vi "canDataSort.vi"() -> ()   [LabVIEW 2023] (continued)
database", "NameShort"="BMS06BattMinTempPoint2", "StartBit"=16, "NumBits"=8, "Min"=-40.0, "Max"=210.0, "ScaleFac"=1.0, "ScaleOff"=-40.0}, {"18F142F3", "Frame"="BMS06\ndatabase", "NameShort"="BMS06BattMinTempPoint2BoxNum", "StartBit"=24, "NumBits"=8, "Min"=0.0, "Max"=100.0, "ScaleFac"=1.0, "ScaleOff"=0.0}, {"18F142F3", "Frame"="BMS06\ndatabase", "NameShort"="BMS06BattMinTempPoint3", "StartBit"=32, "NumBits"=8, "Min"=-40.0, "Max"=210.0, "ScaleFac"=1.0, "ScaleOff"=-40.0}, {"18F142F3", "Frame"="BMS06\ndatabase", "NameShort"="BMS06BattMinTempPoint3BoxNum", "StartBit"=40, "NumBits"=8, "Min"=0.0, "Max"=100.0, "ScaleFac"=1.0, "ScaleOff"=0.0}, {"18F142F3", "Frame"="BMS06\ndatabase", "NameShort"="BMS06BattMinTempPoint4", "StartBit"=48, "NumBits"=8, "Min"=-40.0, "Max"=210.0, "ScaleFac"=1.0, "ScaleOff"=-40.0}, {"18F142F3", "Frame"="BMS06\ndatabase", "NameShort"="BMS06BattMinTempPoint4BoxNum", "StartBit"=56, "NumBits"=8, "Min"=0.0, "Max"=100.0, "ScaleFac"=1.0, "ScaleOff"=0.0}, {"18F143F3", "Frame"="BMS07\ndatabase", "NameShort"="BMS06BattMaxTempPoint1", "StartBit"=0, "NumBits"=8, "Min"=-40.0, "Max"=210.0, "ScaleFac"=1.0, "ScaleOff"=-40.0}, {"18F143F3", "Frame"="BMS07\ndatabase", "NameShort"="BMS06BattMaxTempPoint1BoxNum", "StartBit"=8, "NumBits"=8, "Min"=0.0, "Max"=100.0, "ScaleFac"=1.0, "ScaleOff"=0.0}, {"18F143F3", "Frame"="BMS07\ndatabase", "NameShort"="BMS06BattMaxTempPoint2", "StartBit"=16, "NumBits"=8, "Min"=-40.0, "Max"=210.0, "ScaleFac"=1.0, "ScaleOff"=-40.0}, {"18F143F3", "Frame"="BMS07\ndatabase", "NameShort"="BMS06BattMaxTempPoint2BoxNum", "StartBit"=24, "NumBits"=8, "Min"=0.0, "Max"=100.0, "ScaleFac"=1.0, "ScaleOff"=0.0}, {"18F143F3", "Frame"="BMS07\ndatabase", "NameShort"="BMS06BattMaxTempPoint3", "StartBit"=32, "NumBits"=8, "Min"=-40.0, "Max"=210.0, "ScaleFac"=1.0, "ScaleOff"=-40.0}, {"18F143F3", "Frame"="BMS07\ndatabase", "NameShort"="BMS06BattMaxTempPoint3BoxNum", "StartBit"=40, "NumBits"=8, "Min"=0.0, "Max"=100.0, "ScaleFac"=1.0, "ScaleOff"=0.0}, {"18F143F3", "Frame"="BMS07\ndatabase", "NameShort"="BMS06BattMaxTempPoint4", "StartBit"=48, "NumBits"=8, "Min"=-40.0, "Max"=210.0, "ScaleFac"=1.0, "ScaleOff"=-40.0}, {"18F143F3", "Frame"="BMS07\ndatabase", "NameShort"="BMS06BattMaxTempPoint4BoxNum", "StartBit"=56, "NumBits"=8, "Min"=0.0, "Max"=100.0, "ScaleFac"=1.0, "ScaleOff"=0.0}, {"18F144F3", "Frame"="BMS08\ndatabase", "NameShort"="BMS08BattCellMinVolt1", "StartBit"=0, "NumBits"=16, "Min"=0.0, "Max"=655.35, "ScaleFac"=0.01, "ScaleOff"=0.0}, {"18F144F3", "Frame"="BMS08\ndatabase", "NameShort"="BMS08BattCellMinVolt1Box", "StartBit"=24, "NumBits"=8, "Min"=0.0, "Max"=255.0, "ScaleFac"=1.0, "ScaleOff"=0.0}, {"18F144F3", "Frame"="BMS08\ndatabase", "NameShort"="BMS08BattCellMinVolt1Num", "StartBit"=16, "NumBits"=8, "Min"=0.0, "Max"=100.0, "ScaleFac"=1.0, "ScaleOff"=0.0}, {"18F144F3", "Frame"="BMS08\ndatabase", "NameShort"="BMS08BattCellMinVolt2", "StartBit"=32, "NumBits"=16, "Min"=0.0, "Max"=655.35, "ScaleFac"=0.01, "ScaleOff"=0.0}, {"18F144F3", "Frame"="BMS08\ndatabase", "NameShort"="BMS08BattCellMinVolt2Box", "StartBit"=56, "NumBits"=8, "Min"=0.0, "Max"=255.0, "ScaleFac"=1.0, "ScaleOff"=0.0}, {"18F144F3", "Frame"="BMS08\ndatabase", "NameShort"="BMS08BattCellMinVolt2Num", "StartBit"=48, "NumBits"=8, "Min"=0.0, "Max"=100.0, "ScaleFac"=1.0, "ScaleOff"=0.0}, {"18F145F3", "Frame"="BMS09\ndatabase", "NameShort"="BMS09BattCellMinVolt3", "StartBit"=0, "NumBits"=16, "Min"=0.0, "Max"=655.35, "ScaleFac"=0.01, "ScaleOff"=0.0}, {"18F145F3", "Frame"="BMS09\ndatabase", "NameShort"="BMS09BattCellMinVolt3Box", "StartBit"=24, "NumBits"=8, "Min"=0.0, "Max"=255.0, "ScaleFac"=1.0, "ScaleOff"=0.0}, {"18F145F3", "Frame"="BMS09\ndatabase", "NameShort"="BMS09BattCellMinVolt3Num", "StartBit"=16, "NumBits"=8, "Min"=0.0, "Max"=100.0, "ScaleFac"=1.0, "ScaleOff"=0.0}, {"18F145F3", "Frame"="BMS09\ndatabase", "NameShort"="BMS09BattCellMinVolt4", "StartBit"=32, "NumBits"=16, "Min"=0.0, "Max"=655.35, "ScaleFac"=0.01, "ScaleOff"=0.0}, {"18F145F3", "Frame"="BMS09\ndatabase", "NameShort"="BMS09BattCellMinVolt4Box", "StartBit"=56, "NumBits"=8, "Min"=0.0, "Max"=255.0, "ScaleFac"=1.0, "ScaleOff"=0.0}, {"18F145F3", "Frame"="BMS09\ndatabase", "NameShort"="BMS09BattCellMinVolt4Num", "StartBit"=48, "NumBits"=8, "Min"=0.0, "Max"=100.0, "ScaleFac"=1.0, "ScaleOff"=0.0}, {"18F146F3", "Frame"="BMS10\ndatabase", "NameShort"="BMS10BattCellMinVolt1", "StartBit"=0, "NumBits"=16, "Min"=0.0, "Max"=655.35, "ScaleFac"=0.01, "ScaleOff"=0.0}, {"18F146F3", "Frame"="BMS10\ndatabase", "NameShort"="BMS10BattCellMinVolt1Box", "StartBit"=24, "NumBits"=8, "Min"=0.0, "Max"=255.0, "ScaleFac"=1.0, "ScaleOff"=0.0}, {"18F146F3", "Frame"="BMS10\ndatabase", "NameShort"="BMS10BattCellMinVolt1Num", "StartBit"=16, "NumBits"=8, "Min"=0.0, "Max"=100.0, "ScaleFac"=1.0, "ScaleOff"=0.0}, {"18F146F3", "Frame"="BMS10\ndatabase", "NameShort"="BMS10BattCellMinVolt2", "StartBit"=32, "NumBits"=16, "Min"=0.0, "Max"=655.35, "ScaleFac"=0.01, "ScaleOff"=0.0}, {"18F146F3", "Frame"="BMS10\ndatabase", "NameShort"="BMS10BattCellMinVolt2Box", "StartBit"=56, "NumBits"=8, "Min"=0.0, "Max"=255.0, "ScaleFac"=1.0, "ScaleOff"=0.0}, {"18F146F3", "Frame"="BMS10\ndatabase", "NameShort"="BMS10BattCellMinVolt2Num", "StartBit"=48, "NumBits"=8, "Min"=0.0, "Max"=100.0, "ScaleFac"=1.0, "ScaleOff"=0.0}, {"18F147F3", "Frame"="BMS11\ndatabase", "NameShort"="BMS11BattCellMinVolt3", "StartBit"=0, "NumBits"=16, "Min"=0.0, "Max"=655.35, "ScaleFac"=0.01, "ScaleOff"=0.0}, {"18F147F3", "Frame"="BMS11\ndatabase", "NameShort"="BMS11BattCellMinVolt3Box", "StartBit"=24, "NumBits"=8, "Min"=0.0, "Max"=255.0, "ScaleFac"=1.0, "ScaleOff"=0.0}, {"18F147F3", "Frame"="BMS11\ndatabase", "NameShort"="BMS11BattCellMinVolt3Num", "StartBit"=16, "NumBits"=8, "Min"=0.0, "Max"=100.0, "ScaleFac"=1.0, "ScaleOff"=0.0}, {"18F147F3", "Frame"="BMS11\ndatabase", "NameShort"="BMS11BattCellMinVolt4", "StartBit"=32, "NumBits"=16, "Min"=0.0, "Max"=655.35, "ScaleFac"=0.01, "ScaleOff"=0.0}, {"18F147F3", "Frame"="BMS11\ndatabase", "NameShort"="BMS11BattCellMinVolt4Box", "StartBit"=56, "NumBits"=8, "Min"=0.0, "Max"=255.0, "ScaleFac"=1.0, "ScaleOff"=0.0}, {"18F147F3", "Frame"="BMS11\ndatabase", "NameShort"="BMS11BattCellMinVolt4Num", "StartBit"=48, "NumBits"=8, "Min"=0.0, "Max"=100.0, "ScaleFac"=1.0, "ScaleOff"=0.0}, {"18F148F3", "Frame"="BMS12\ndatabase", "NameShort"="BMS12BattPackProdMonth", "StartBit"=40, "NumBits"=8, "Min"=0.0, "Max"=12.0, "ScaleFac"=1.0, "ScaleOff"=0.0}, {"18F148F3", "Frame"="BMS12\ndatabase", "NameShort"="BMS12BattPackProdYear", "StartBit"=32, "NumBits"=8, "Min"=1985.0, "Max"=2235.0, "ScaleFac"=1.0, "ScaleOff"=1985.0}, {"18F148F3", "Frame"="BMS12\ndatabase", "NameShort"="BMS12BattProdDay", "StartBit"=48, "NumBits"=8, "Min"=0.0, "Max"=31.0, "ScaleFac"=1.0, "ScaleOff"=0.0}, {"18F148F3", "Frame"="BMS12\ndatabase", "NameShort"="BMS12BattRatedCapacity", "StartBit"=0, "NumBits"=16, "Min"=0.0, "Max"=1000.0, "ScaleFac"=1.0, "ScaleOff"=0.0}, {"18F148F3", "Frame"="BMS12\ndatabase", "NameShort"="BMS12BattRatedVolt", "StartBit"=16, "NumBits"=16, "Min"=0.0, "Max"=1000.0, "ScaleFac"=1.0, "ScaleOff"=0.0}, {"18FFC3A9", "Frame"="BluestarAirConErrorNBoot\ndatabase", "NameShort"="BluestarAirConElectricBoxPow", "StartBit"=40, "NumBits"=2, "Min"=0.0, "Max"=2.0, "ScaleFac"=1.0, "ScaleOff"=0.0}, {"18FFC3A9", "Frame"="BluestarAirConErrorNBoot\ndatabase", "NameShort"="BluestarAirConErr01Overvoltage", "StartBit"=4, "NumBits"=2, "Min"=0.0, "Max"=1.0, "ScaleFac"=1.0, "ScaleOff"=0.0}, {"18FFC3A9", "Frame"="BluestarAirConErrorNBoot\ndatabase", "NameShort"="BluestarAirConErr02Undervoltage", "StartBit"=6, "NumBits"=2, "Min"=0.0, "Max"=1.0, "ScaleFac"=1.0, "ScaleOff"=0.0}, {"18FFC3A9", "Frame"="BluestarAirConErrorNBoot\ndatabase", "NameShort"="BluestarAirConErr03UnderPressure", "StartBit"=0, "NumBits"=2, "Min"=0.0, "Max"=2.0, "ScaleFac"=1.0, "ScaleOff"=0.0}, {"18FFC3A9", "Frame"="BluestarAirConErrorNBoot\ndatabase", "NameShort"="BluestarAirConErr04EDefroster", "StartBit"=14, "NumBits"=2, "Min"=0.0, "Max"=2.0, "ScaleFac"=1.0, "ScaleOff"=0.0}, {"18FFC3A9", "Frame"="BluestarAirConErrorNBoot\ndatabase", "NameShort"="BluestarAirConErr05IndoorSensor", "StartBit"=8, "NumBits"=2, "Min"=0.0, "Max"=2.0, "ScaleFac"=1.0, "ScaleOff"=0.0}, {"18FFC3A9", "Frame"="BluestarAirConErrorNBoot\ndatabase", "NameShort"="BluestarAirConErr07OverPressure", "StartBit"=2, "NumBits"=2, "Min"=0.0, "Max"=2.0, "ScaleFac"=1.0, "ScaleOff"=0.0}, {"18FFC3A9", "Frame"="BluestarAirConErrorNBoot\ndatabase", "NameShort"="BluestarAirConErr08OutdoorSensor", "StartBit"=10, "NumBits"=2, "Min"=0.0, "Max"=2.0, "ScaleFac"=1.0, "ScaleOff"=0.0}, {"18FFC3A9", "Frame"="BluestarAirConErrorNBoot\ndatabase", "NameShort"="BluestarAirConErr09Compressor", "StartBit"=32, "NumBits"=2, "Min"=0.0, "Max"=2.0, "ScaleFac"=1.0, "ScaleOff"=0.0}, {"18FFC3A9", "Frame"="BluestarAirConErrorNBoot\ndatabase", "NameShort"="BluestarAirConErr10Inverter", "StartBit"=28, "NumBits"=2, "Min"=0.0, "Max"=2.0, "ScaleFac"=1.0, "ScaleOff"=0.0}, {"18FFC2A9", "Frame"="BluestarAirConRemotePowerContro2\ndatabase", "NameShort"="BluestarAirConIndoorTemp", "StartBit"=0, "NumBits"=8, "Min"=-40.0, "Max"=210.0, "ScaleFac"=1.0, "ScaleOff"=-40.0}, {"18FFC2A9", "Frame"="BluestarAirConRemotePowerContro2\ndatabase", "NameShort"="BluestarAirConOutdoorTemp", "StartBit"=8, "NumBits"=8, "Min"=-40.0, "Max"=210.0, "ScaleFac"=1.0, "ScaleOff"=-40.0}, {"18FFC1A8", "Frame"="BluestarAirConRemotePowerControl\ndatabase", "NameShort"="BluestarAirConAutoMode", "StartBit"=44, "NumBits"=2, "Min"=0.0, "Max"=1.0, "ScaleFac"=1.0, "ScaleOff"=0.0}, {"18FFC1A8", "Frame"="BluestarAirConRemotePowerControl\ndatabase", "NameShort"="BluestarAirConFanSpeed", "StartBit"=4, "NumBits"=4, "Min"=0.0, "Max"=1.0, "ScaleFac"=1.0, "ScaleOff"=0.0}, {"18FFC1A8", "Frame"="BluestarAirConRemotePowerControl\ndatabase", "NameShort"="BluestarAirConMode", "StartBit"=8, "NumBits"=8, "Min"=0.0, "Max"=1.0, "ScaleFac"=1.0, "ScaleOff"=0.0}, {"18FFC1A8", "Frame"="BluestarAirConRemotePowerControl\ndatabase", "NameShort"="BluestarAirConPowerOnOff", "StartBit"=0, "NumBits"=2, "Min"=0.0, "Max"=1.0, "ScaleFac"=1.0, "ScaleOff"=0.0}, {"18FFC1A8", "Frame"="BluestarAirConRemotePowerControl\ndatabase", "NameShort"="BluestarAirConSetTemp", "StartBit"=16, "NumBits"=8, "Min"=-40.0, "Max"=210.0, "ScaleFac"=1.0, "ScaleOff"=-40.0}, {"142CFF98", "Frame"="DCDC\ndatabase", "NameShort"="DCDCErrCode", "StartBit"=56, "NumBits"=4, "Min"=0.0, "Max"=15.0, "ScaleFac"=1.0, "ScaleOff"=0.0}, {"142CFF98", "Frame"="DCDC\ndatabase", "NameShort"="DCDCINCurr", "StartBit"=16, "NumBits"=8, "Min"=0.0, "Max"=100.0, "ScaleFac"=1.0, "ScaleOff"=0.0}, {"142CFF98", "Frame"="DCDC\ndatabase", "NameShort"="DCDCINVolt", "StartBit"=0, "NumBits"=16, "Min"=0.0, "Max"=1000.0, "ScaleFac"=0.1, "ScaleOff"=0.0}, {"142CFF98", "Frame"="DCDC\ndatabase", "NameShort"="DCDCLife", "StartBit"=48, "NumBits"=8, "Min"=0.0, "Max"=255.0, "ScaleFac"=1.0, "ScaleOff"=0.0}, {"142CFF98", "Frame"="DCDC\ndatabase", "NameShort"="DCDCOUTCurr", "StartBit"=24, "NumBits"=8, "Min"=0.0, "Max"=100.0, "ScaleFac"=1.0, "ScaleOff"=0.0}, {"142CFF98", "Frame"="DCDC\ndatabase", "NameShort"="DCDCOUTVolt", "StartBit"=40, "NumBits"=8, "Min"=0.0, "Max"=100.0, "ScaleFac"=1.0, "ScaleOff"=0.0}, {"142CFF98", "Frame"="DCDC\ndatabase", "NameShort"="DCDCPrechgStat", "StartBit"=63, "NumBits"=1, "Min"=0.0, "Max"=1.0, "ScaleFac"=1.0, "ScaleOff"=0.0}, {"142CFF98", "Frame"="DCDC\ndatabase", "NameShort"="DCDCStat", "StartBit"=60, "NumBits"=2, "Min"=0.0, "Max"=1.0, "ScaleFac"=1.0, "ScaleOff"=0.0}, {"142CFF98", "Frame"="DCDC\ndatabase", "NameShort"="DCDCTemp", "StartBit"=32, "NumBits"=8, "Min"=-40.0, "Max"=200.0, "ScaleFac"=1.0, "ScaleOff"=-40.0}, {"142CFF97", "Frame"="DCDC2\ndatabase", "NameShort"="DCDC2ErrCode", "StartBit"=56, "NumBits"=4, "Min"=0.0, "Max"=15.0, "ScaleFac"=1.0, "ScaleOff"=0.0}, {"142CFF97", "Frame"="DCDC2\ndatabase", "NameShort"="DCDC2INCurr", "StartBit"=16, "NumBits"=8, "Min"=0.0, "Max"=100.0, "ScaleFac"=1.0, "ScaleOff"=0.0}, {"142CFF97", "Frame"="DCDC2\ndatabase", "NameShort"="DCDC2INVolt", "StartBit"=0, "NumBits"=16, "Min"=0.0, "Max"=1000.0, "ScaleFac"=0.1, "ScaleOff"=0.0}, {"142CFF97", "Frame"="DCDC2\ndatabase", "NameShort"="DCDC2Life", "StartBit"=48, "NumBits"=8, "Min"=0.0, "Max"=255.0, "ScaleFac"=1.0, "ScaleOff"=0.0}, {"142CFF97", "Frame"="DCDC2\ndatabase", "NameShort"="DCDC2OUTCurr", "StartBit"=24, "NumBits"=8, "Min"=0.0, "Max"=100.0, "ScaleFac"=1.0, "ScaleOff"=0.0}, {"142CFF97", "Frame"="DCDC2\ndatabase", "NameShort"="DCDC2OUTVolt", "StartBit"=40, "NumBits"=8, "Min"=0.0, "Max"=100.0, "ScaleFac"=1.0, "ScaleOff"=0.0}, {"142CFF97", "Frame"="DCDC2\ndatabase", "NameShort"="DCDC2PrechgStat", "StartBit"=63, "NumBits"=1, "Min"=0.0, "Max"=1.0, "ScaleFac"=1.0, "ScaleOff"=0.0}, {"142CFF97", "Frame"="DCDC2\ndatabase", "NameShort"="DCDC2Stat", "StartBit"=60, "NumBits"=2, "Min"=0.0, "Max"=1.0, "ScaleFac"=1.0, "ScaleOff"=0.0}, {"142CFF97", "Frame"="DCDC2\ndatabase", "NameShort"="DCDC2Temp", "StartBit"=32, "NumBits"=8, "Min"=-40.0, "Max"=200.0, "ScaleFac"=1.0, "ScaleOff"=-40.0}, {"142FFF95", "Frame"="Ehps1\ndatabase", "NameShort"="Ehps1Curr", "StartBit"=32, "NumBits"=8, "Min"=0.0, "Max"=100.0, "ScaleFac"=1.0, "ScaleOff"=0.0}, {"142FFF95", "Frame"="Ehps1\ndatabase", "NameShort"="Ehps1Life", "StartBit"=48, "NumBits"=8, "Min"=0.0, "Max"=255.0, "ScaleFac"=1.0, "ScaleOff"=0.0}, {"142FFF95", "Frame"="Ehps1\ndatabase", "NameShort"="Ehps1MalfuncCode1", "StartBit"=56, "NumBits"=4, "Min"=0.0, "Max"=15.0, "ScaleFac"=1.0, "ScaleOff"=0.0}, {"142FFF95", "Frame"="Ehps1\ndatabase", "NameShort"="Ehps1MtrSpeed", "StartBit"=0, "NumBits"=16, "Min"=0.0, "Max"=5000.0, "ScaleFac"=0.125, "ScaleOff"=0.0}, {"142FFF95", "Frame"="Ehps1\ndatabase", "NameShort"="Ehps1OilPumpStat", "StartBit"=60, "NumBits"=2, "Min"=0.0, "Max"=1.0, "ScaleFac"=1.0, "ScaleOff"=0.0}, {"142FFF95", "Frame"="Ehps1\ndatabase", "NameShort"="Ehps1PreChgStat", "StartBit"=63, "NumBits"=1, "Min"=0.0, "Max"=1.0, "ScaleFac"=1.0, "ScaleOff"=0.0}, {"142FFF95", "Frame"="Ehps1\ndatabase", "NameShort"="Ehps1Stat", "StartBit"=62, "NumBits"=1, "Min"=0.0, "Max"=1.0, "ScaleFac"=1.0, "ScaleOff"=0.0}, {"142FFF95", "Frame"="Ehps1\ndatabase", "NameShort"="Ehps1Temp", "StartBit"=40, "NumBits"=8, "Min"=-40.0, "Max"=210.0, "ScaleFac"=1.0, "ScaleOff"=-40.0}, {"142FFF95", "Frame"="Ehps1\ndatabase", "NameShort"="Ehps1Volt", "StartBit"=16, "NumBits"=16, "Min"=0.0, "Max"=1000.0, "ScaleFac"=0.1, "ScaleOff"=0.0}, {"18FFA7A9", "Frame"="FiveInOne\ndatabase", "NameShort"="FiveInOneAirComprRelayStat", "StartBit"=14, "NumBits"=2, "Min"=0.0, "Max"=1.0, "ScaleFac"=1.0, "ScaleOff"=0.0}, {"18FFA7A9", "Frame"="FiveInOne\ndatabase", "NameShort"="FiveInOneAirConRelayStat", "StartBit"=12, "NumBits"=2, "Min"=0.0, "Max"=1.0, "ScaleFac"=1.0, "ScaleOff"=0.0}, {"18FFA7A9", "Frame"="FiveInOne\ndatabase", "NameShort"="FiveInOneBrkResistRelayStat", "StartBit"=24, "NumBits"=2, "Min"=0.0, "Max"=1.0, "ScaleFac"=1.0, "ScaleOff"=0.0}, {"18FFA7A9", "Frame"="FiveInOne\ndatabase", "NameShort"="FiveInOneDCDCRelayStat", "StartBit"=2, "NumBits"=2, "Min"=0.0, "Max"=1.0, "ScaleFac"=1.0, "ScaleOff"=0.0}, {"18FFA7A9", "Frame"="FiveInOne\ndatabase", "NameShort"="FiveInOneDefrostRelayStat", "StartBit"=10, "NumBits"=2, "Min"=0.0, "Max"=1.0, "ScaleFac"=1.0, "ScaleOff"=0.0}, {"18FFA7A9", "Frame"="FiveInOne\ndatabase", "NameShort"="FiveInOneEHPSRelayStat", "StartBit"=0, "NumBits"=2, "Min"=0.0, "Max"=1.0, "ScaleFac"=1.0, "ScaleOff"=0.0}, {"18FFA7A9", "Frame"="FiveInOne\ndatabase", "NameShort"="FiveInOneHeaterRelayStat", "StartBit"=22, "NumBits"=2, "Min"=0.0, "Max"=1.0, "ScaleFac"=1.0, "ScaleOff"=0.0}, {"18FFA7A9", "Frame"="FiveInOne\ndatabase", "NameShort"="FiveInOneLife", "StartBit"=56, "NumBits"=8, "Min"=0.0, "Max"=255.0, "ScaleFac"=1.0, "ScaleOff"=0.0}, {"18FFA7A9", "Frame"="FiveInOne\ndatabase", "NameShort"="FiveInOneMtrRelayStat", "StartBit"=4, "NumBits"=2, "Min"=0.0, "Max"=1.0, "ScaleFac"=1.0, "ScaleOff"=0.0}, {"18FFA7A9", "Frame"="FiveInOne\ndatabase", "NameShort"="FiveInOnePluginStat", "StartBit"=8, "NumBits"=2, "Min"=0.0, "Max"=1.0, "ScaleFac"=1.0, "ScaleOff"=0.0}, {"18FFA7A9", "Frame"="FiveInOne\ndatabase", "NameShort"="FiveInOnePrechgRelayStat", "StartBit"=6, "NumBits"=2, "Min"=0.0, "Max"=1.0, "ScaleFac"=1.0, "ScaleOff"=0.0}, {"1801D0A7", "Frame"="INVTDCDCStat\ndatabase", "NameShort"="INVTDCDCFaultLvl", "StartBit"=8, "NumBits"=2, "Min"=0.0, "Max"=3.0, "ScaleFac"=1.0, "ScaleOff"=0.0}, {"1801D0A7", "Frame"="INVTDCDCStat\ndatabase", "NameShort"="INVTDCDCStatErrCode", "StartBit"=0, "NumBits"=8, "Min"=0.0, "Max"=255.0, "ScaleFac"=1.0, "ScaleOff"=0.0}, {"1801D0A7", "Frame"="INVTDCDCStat\ndatabase", "NameShort"="INVTDCDCStatFaultStat", "StartBit"=14, "NumBits"=2, "Min"=0.0, "Max"=3.0, "ScaleFac"=1.0, "ScaleOff"=0.0}, {"1801D0A7", "Frame"="INVTDCDCStat\ndatabase", "NameShort"="INVTDCDCStatINCurr", "StartBit"=32, "NumBits"=16, "Min"=0.0, "Max"=6553.5, "ScaleFac"=0.1, "ScaleOff"=0.0}, {"1801D0A7", "Frame"="INVTDCDCStat\ndatabase", "NameShort"="INVTDCDCStatINVolt", "StartBit"=16, "NumBits"=16, "Min"=0.0, "Max"=1000.0, "ScaleFac"=0.1, "ScaleOff"=0.0}, {"1801D0A7", "Frame"="INVTDCDCStat\ndatabase", "NameShort"="INVTDCDCStatLife", "StartBit"=56, "NumBits"=8, "Min"=0.0, "Max"=255.0, "ScaleFac"=1.0, "ScaleOff"=0.0}, {"1801D0A7", "Frame"="INVTDCDCStat\ndatabase", "NameShort"="INVTDCDCStatPowerStat", "StartBit"=10, "NumBits"=2, "Min"=0.0, "Max"=3.0, "ScaleFac"=1.0, "ScaleOff"=0.0}, {"1801D0A7", "Frame"="INVTDCDCStat\ndatabase", "NameShort"="INVTDCDCStatTemp", "StartBit"=48, "NumBits"=8, "Min"=-40.0, "Max"=200.0, "ScaleFac"=1.0, "ScaleOff"=-40.0}, {"1801D0A7", "Frame"="INVTDCDCStat\ndatabase", "NameShort"="INVTDCDCStatWorkStat", "StartBit"=12, "NumBits"=2, "Min"=0.0, "Max"=3.0, "ScaleFac"=1.0, "ScaleOff"=0.0}, {"1802D0A7", "Frame"="INVTDCDCStat2\ndatabase", "NameShort"="INVTDCDCStat2OUTCurr", "StartBit"=16, "NumBits"=16, "Min"=0.0, "Max"=500.0, "ScaleFac"=0.1, "ScaleOff"=0.0}, {"1802D0A7", "Frame"="INVTDCDCStat2\ndatabase", "NameShort"="INVTDCDCStat2OUTVolt", "StartBit"=0, "NumBits"=16, "Min"=0.0, "Max"=1000.0, "ScaleFac"=0.1, "ScaleOff"=0.0}, {"1801D0A6", "Frame"="INVTEACStat\ndatabase", "NameShort"="INVTEACFaultLvl", "StartBit"=8, "NumBits"=2, "Min"=0.0, "Max"=3.0, "ScaleFac"=1.0, "ScaleOff"=0.0}, {"1801D0A6", "Frame"="INVTEACStat\ndatabase", "NameShort"="INVTEACStatErrCode", "StartBit"=0, "NumBits"=8, "Min"=0.0, "Max"=255.0, "ScaleFac"=1.0, "ScaleOff"=0.0}, {"1801D0A6", "Frame"="INVTEACStat\ndatabase", "NameShort"="INVTEACStatFaultStat", "StartBit"=14, "NumBits"=2, "Min"=0.0, "Max"=3.0, "ScaleFac"=1.0, "ScaleOff"=0.0}, {"1801D0A6", "Frame"="INVTEACStat\ndatabase", "NameShort"="INVTEACStatINVolt", "StartBit"=16, "NumBits"=16, "Min"=0.0, "Max"=1000.0, "ScaleFac"=0.1, "ScaleOff"=0.0}, {"1801D0A6", "Frame"="INVTEACStat\ndatabase", "NameShort"="INVTEACStatInvertorTemp", "StartBit"=48, "NumBits"=8, "Min"=-40.0, "Max"=150.0, "ScaleFac"=1.0, "ScaleOff"=-40.0}, {"1801D0A6", "Frame"="INVTEACStat\ndatabase", "NameShort"="INVTEACStatLife", "StartBit"=56, "NumBits"=8, "Min"=0.0, "Max"=255.0, "ScaleFac"=1.0, "ScaleOff"=0.0}, {"1801D0A6", "Frame"="INVTEACStat\ndatabase", "NameShort"="INVTEACStatMtrTemp", "StartBit"=32, "NumBits"=8, "Min"=-40.0, "Max"=200.0, "ScaleFac"=1.0, "ScaleOff"=-40.0}, {"1801D0A6", "Frame"="INVTEACStat\ndatabase", "NameShort"="INVTEACStatPowerStat", "StartBit"=10, "NumBits"=2, "Min"=0.0, "Max"=3.0, "ScaleFac"=1.0, "ScaleOff"=0.0}, {"1801D0A6", "Frame"="INVTEACStat\ndatabase", "NameShort"="INVTEACStatWorkStat", "StartBit"=12, "NumBits"=2, "Min"=0.0, "Max"=3.0, "ScaleFac"=1.0, "ScaleOff"=0.0}, {"1802D0A6", "Frame"="INVTEACStat2\ndatabase", "NameShort"="INVTEACStat2INCurr", "StartBit"=48, "NumBits"=16, "Min"=0.0, "Max"=6553.5, "ScaleFac"=0.1, "ScaleOff"=0.0}, {"1802D0A6", "Frame"="INVTEACStat2\ndatabase", "NameShort"="INVTEACStat2Mtrrpm", "StartBit"=0, "NumBits"=16, "Min"=-5000.0, "Max"=5000.0, "ScaleFac"=0.5, "ScaleOff"=-5000.0}, {"1802D0A6", "Frame"="INVTEACStat2\ndatabase", "NameShort"="INVTEACStat2OUTCurr", "StartBit"=32, "NumBits"=16, "Min"=0.0, "Max"=500.0, "ScaleFac"=0.1, "ScaleOff"=0.0}, {"1802D0A6", "Frame"="INVTEACStat2\ndatabase", "NameShort"="INVTEACStat2OUTVolt", "StartBit"=16, "NumBits"=16, "Min"=0.0, "Max"=1000.0, "ScaleFac"=0.1, "ScaleOff"=0.0}, {"1801D0A5", "Frame"="INVTEHPSStat\ndatabase", "NameShort"="INVTEHPSFaultLvl", "StartBit"=8, "NumBits"=2, "Min"=0.0, "Max"=3.0, "ScaleFac"=1.0, "ScaleOff"=0.0}, {"1801D0A5", "Frame"="INVTEHPSStat\ndatabase", "NameShort"="INVTEHPSStatErrCode", "StartBit"=0, "NumBits"=8, "Min"=0.0, "Max"=255.0, "ScaleFac"=1.0, "ScaleOff"=0.0}, {"1801D0A5", "Frame"="INVTEHPSStat\ndatabase", "NameShort"="INVTEHPSStatFaultStat", "StartBit"=14, "NumBits"=2, "Min"=0.0, "Max"=3.0, "ScaleFac"=1.0, "ScaleOff"=0.0}, {"1801D0A5", "Frame"="INVTEHPSStat\ndatabase", "NameShort"="INVTEHPSStatINVolt", "StartBit"=16, "NumBits"=16, "Min"=0.0, "Max"=1000.0, "ScaleFac"=0.1, "ScaleOff"=0.0}, {"1801D0A5", "Frame"="INVTEHPSStat\ndatabase", "NameShort"="INVTEHPSStatInvertorTemp", "StartBit"=48, "NumBits"=8, "Min"=-40.0, "Max"=150.0, "ScaleFac"=1.0, "ScaleOff"=-40.0}, {"1801D0A5", "Frame"="INVTEHPSStat\ndatabase", "NameShort"="INVTEHPSStatLife", "StartBit"=56, "NumBits"=8, "Min"=0.0, "Max"=255.0, "ScaleFac"=1.0, "ScaleOff"=0.0}, {"1801D0A5", "Frame"="INVTEHPSStat\ndatabase", "NameShort"="INVTEHPSStatMtrTemp", "StartBit"=32, "NumBits"=8, "Min"=-40.0, "Max"=200.0, "ScaleFac"=1.0, "ScaleOff"=-40.0}, {"1801D0A5", "Frame"="INVTEHPSStat\ndatabase", "NameShort"="INVTEHPSStatPowerStat", "StartBit"=10, "NumBits"=2, "Min"=0.0, "Max"=3.0, "ScaleFac"=1.0, "ScaleOff"=0.0}, {"1801D0A5", "Frame"="INVTEHPSStat\ndatabase", "NameShort"="INVTEHPSStatWorkStat", "StartBit"=12, "NumBits"=2, "Min"=0.0, "Max"=3.0, "ScaleFac"=1.0, "ScaleOff"=0.0}, {"1802D0A5", "Frame"="INVTEHPSStat2\ndatabase", "NameShort"="INVTEHPSStat2INCurr", "StartBit"=48, "NumBits"=16, "Min"=0.0, "Max"=6553.5, "ScaleFac"=0.1, "ScaleOff"=0.0}, {"1802D0A5", "Frame"="INVTEHPSStat2\ndatabase", "NameShort"="INVTEHPSStat2Mtrrpm", "StartBit"=0, "NumBits"=16, "Min"=-5000.0, "Max"=5000.0, "ScaleFac"=0.5, "ScaleOff"=-5000.0}, {"1802D0A5", "Frame"="INVTEHPSStat2\ndatabase", "NameShort"="INVTEHPSStat2OUTCurr", "StartBit"=32, "NumBits"=16, "Min"=0.0, "Max"=500.0, "ScaleFac"=0.1, "ScaleOff"=0.0}, {"1802D0A5", "Frame"="INVTEHPSStat2\ndatabase", "NameShort"="INVTEHPSStat2OUTVolt", "StartBit"=16, "NumBits"=16, "Min"=0.0, "Max"=1000.0, "ScaleFac"=0.1, "ScaleOff"=0.0}, {"1801D0D7", "Frame"="INVTInsulationTester\ndatabase", "NameShort"="INVTInsulationTestErrorLv", "StartBit"=32, "NumBits"=8, "Min"=0.0, "Max"=255.0, "ScaleFac"=1.0, "ScaleOff"=0.0}, {"1801D0D7", "Frame"="INVTInsulationTester\ndatabase", "NameShort"="INVTInsulationTestLife", "StartBit"=40, "NumBits"=8, "Min"=0.0, "Max"=255.0, "ScaleFac"=1.0, "ScaleOff"=0.0}, {"1801D0D7", "Frame"="INVTInsulationTester\ndatabase", "NameShort"="INVTInsulationTestNEGtoGNDResist", "StartBit"=16, "NumBits"=16, "Min"=0.0, "Max"=65535.0, "ScaleFac"=1.0, "ScaleOff"=0.0}, {"1801D0D7", "Frame"="INVTInsulationTester\ndatabase", "NameShort"="INVTInsulationTestPOStoGNDResist", "StartBit"=0, "NumBits"=16, "Min"=0.0, "Max"=65535.0, "ScaleFac"=1.0, "ScaleOff"=0.0}, {"1801D0D7", "Frame"="INVTInsulationTester\ndatabase", "NameShort"="INVTInsulationTestStat", "StartBit"=48, "NumBits"=8, "Min"=0.0, "Max"=255.0, "ScaleFac"=1.0, "ScaleOff"=0.0}, {"18F301A8", "Frame"="INVTPDU\ndatabase", "NameShort"="INVTPDUACHVLoopStat", "StartBit"=26, "NumBits"=2, "Min"=0.0, "Max"=3.0, "ScaleFac"=1.0, "ScaleOff"=0.0}, {"18F301A8", "Frame"="INVTPDU\ndatabase", "NameShort"="INVTPDUACPrechrgRlyStat", "StartBit"=20, "NumBits"=2, "Min"=0.0, "Max"=3.0, "ScaleFac"=1.0, "ScaleOff"=0.0}, {"18F301A8", "Frame"="INVTPDU\ndatabase", "NameShort"="INVTPDUACRlyStat", "StartBit"=22, "NumBits"=2, "Min"=0.0, "Max"=3.0, "ScaleFac"=1.0, "ScaleOff"=0.0}, {"18F301A8", "Frame"="INVTPDU\ndatabase", "NameShort"="INVTPDUFaultLvl", "StartBit"=32, "NumBits"=2, "Min"=0.0, "Max"=3.0, "ScaleFac"=1.0, "ScaleOff"=0.0}, {"18F301A8", "Frame"="INVTPDU\ndatabase", "NameShort"="INVTPDULife", "StartBit"=56, "NumBits"=8, "Min"=0.0, "Max"=255.0, "ScaleFac"=1.0, "ScaleOff"=0.0}, {"18F301A8", "Frame"="INVTPDU\ndatabase", "NameShort"="INVTPDUMCUHVLoopStat", "StartBit"=2, "NumBits"=2, "Min"=0.0, "Max"=3.0, "ScaleFac"=1.0, "ScaleOff"=0.0}, {"18F301A8", "Frame"="INVTPDU\ndatabase", "NameShort"="INVTPDUMCUMainRlyStat", "StartBit"=4, "NumBits"=2, "Min"=0.0, "Max"=3.0, "ScaleFac"=1.0, "ScaleOff"=0.0}, {"18F301A8", "Frame"="INVTPDU\ndatabase", "NameShort"="INVTPDUMCUPrechrgRlyStat", "StartBit"=6, "NumBits"=2, "Min"=0.0, "Max"=3.0, "ScaleFac"=1.0, "ScaleOff"=0.0}, {"18F301A8", "Frame"="INVTPDU\ndatabase", "NameShort"="INVTPDUStat", "StartBit"=0, "NumBits"=2, "Min"=0.0, "Max"=3.0, "ScaleFac"=1.0, "ScaleOff"=0.0}, {"18F301B8", "Frame"="INVTPDU2\ndatabase", "NameShort"="INVTPDU2INVolt", "StartBit"=0, "NumBits"=16, "Min"=0.0, "Max"=6553.5, "ScaleFac"=0.1, "ScaleOff"=0.0}, {"18F43A17", "Frame"="IP\ndatabase", "NameShort"="IP24V", "StartBit"=0, "NumBits"=8, "Min"=0.0, "Max"=50.0, "ScaleFac"=0.2, "ScaleOff"=0.0}, {"18F43A17", "Frame"="IP\ndatabase", "NameShort"="IPACCKeyPosnStat", "StartBit"=15, "NumBits"=1, "Min"=0.0, "Max"=1.0, "ScaleFac"=1.0, "ScaleOff"=0.0}, {"18F43A17", "Frame"="IP\ndatabase", "NameShort"="IPFrontAirReservoirPressure", "StartBit"=16, "NumBits"=8, "Min"=0.0, "Max"=1.0, "ScaleFac"=0.01, "ScaleOff"=0.0}, {"18F43A17", "Frame"="IP\ndatabase", "NameShort"="IPFrontDoorStat", "StartBit"=10, "NumBits"=1, "Min"=0.0, "Max"=1.0, "ScaleFac"=1.0, "ScaleOff"=0.0}, {"18F43A17", "Frame"="IP\ndatabase", "NameShort"="IPHandbrkStat", "StartBit"=12, "NumBits"=1, "Min"=0.0, "Max"=1.0, "ScaleFac"=1.0, "ScaleOff"=0.0}, {"18F43A17", "Frame"="IP\ndatabase", "NameShort"="IPHatchDoorStat", "StartBit"=11, "NumBits"=1, "Min"=0.0, "Max"=1.0, "ScaleFac"=1.0, "ScaleOff"=0.0}, {"18F43A17", "Frame"="IP\ndatabase", "NameShort"="IPLife", "StartBit"=56, "NumBits"=8, "Min"=0.0, "Max"=255.0, "ScaleFac"=1.0, "ScaleOff"=0.0}, {"18F43A17", "Frame"="IP\ndatabase", "NameShort"="IPMidDoorStat", "StartBit"=9, "NumBits"=1, "Min"=0.0, "Max"=1.0, "ScaleFac"=1.0, "ScaleOff"=0.0}, {"18F43A17", "Frame"="IP\ndatabase", "NameShort"="IPONKeyPosnStat", "StartBit"=14, "NumBits"=1, "Min"=0.0, "Max"=1.0, "ScaleFac"=1.0, "ScaleOff"=0.0}, {"18F43A17", "Frame"="IP\ndatabase", "NameShort"="IPRearAirReservoirPressure", "StartBit"=24, "NumBits"=8, "Min"=0.0, "Max"=1.0, "ScaleFac"=0.01, "ScaleOff"=0.0}, {"18F43A17", "Frame"="IP\ndatabase", "NameShort"="IPRearDoorStat", "StartBit"=8, "NumBits"=1, "Min"=0.0, "Max"=1.0, "ScaleFac"=1.0, "ScaleOff"=0.0}, {"18F43A17", "Frame"="IP\ndatabase", "NameShort"="IPSmokeDetectStat", "StartBit"=13, "NumBits"=1, "Min"=0.0, "Max"=1.0, "ScaleFac"=1.0, "ScaleOff"=0.0}, {"18F43A17", "Frame"="IP\ndatabase", "NameShort"="IPSpeedLimitReq", "StartBit"=33, "NumBits"=1, "Min"=0.0, "Max"=1.0, "ScaleFac"=1.0, "ScaleOff"=0.0}, {"18F43A17", "Frame"="IP\ndatabase", "NameShort"="IPThrottleInterlockReq", "StartBit"=32, "NumBits"=1, "Min"=0.0, "Max"=1.0, "ScaleFac"=1.0, "ScaleOff"=0.0}, {"18A70017", "Frame"="IP2\ndatabase", "NameShort"="IP2ABSStat", "StartBit"=42, "NumBits"=2, "Min"=0.0, "Max"=3.0, "ScaleFac"=1.0, "ScaleOff"=0.0}, {"18A70017", "Frame"="IP2\ndatabase", "NameShort"="IP2AirConStat", "StartBit"=14, "NumBits"=2, "Min"=0.0, "Max"=3.0, "ScaleFac"=1.0, "ScaleOff"=0.0}, {"18A70017", "Frame"="IP2\ndatabase", "NameShort"="IP2AirFilterClogWarn", "StartBit"=10, "NumBits"=2, "Min"=0.0, "Max"=3.0, "ScaleFac"=1.0, "ScaleOff"=0.0}, {"18A70017", "Frame"="IP2\ndatabase", "NameShort"="IP2BrkPadsWornOutWarn", "StartBit"=8, "NumBits"=2, "Min"=0.0, "Max"=3.0, "ScaleFac"=1.0, "ScaleOff"=0.0}, {"18A70017", "Frame"="IP2\ndatabase", "NameShort"="IP2BrkPressureWarn", "StartBit"=2, "NumBits"=2, "Min"=0.0, "Max"=3.0, "ScaleFac"=1.0, "ScaleOff"=0.0}, {"18A70017", "Frame"="IP2\ndatabase", "NameShort"="IP2BrkStat", "StartBit"=36, "NumBits"=2, "Min"=0.0, "Max"=3.0, "ScaleFac"=1.0, "ScaleOff"=0.0}, {"18A70017", "Frame"="IP2\ndatabase", "NameShort"="IP2EHPSWarn", "StartBit"=4, "NumBits"=2, "Min"=0.0, "Max"=3.0, "ScaleFac"=1.0, "ScaleOff"=0.0}, {"18A70017", "Frame"="IP2\ndatabase", "NameShort"="IP2EngineOilTempWarn", "StartBit"=54, "NumBits"=2, "Min"=0.0, "Max"=3.0, "ScaleFac"=1.0, "ScaleOff"=0.0}, {"18A70017", "Frame"="IP2\ndatabase", "NameShort"="IP2FogLightSig", "StartBit"=26, "NumBits"=2, "Min"=0.0, "Max"=3.0, "ScaleFac"=1.0, "ScaleOff"=0.0}, {"18A70017", "Frame"="IP2\ndatabase", "NameShort"="IP2FrontDoorSig", "StartBit"=20, "NumBits"=2, "Min"=0.0, "Max"=3.0, "ScaleFac"=1.0, "ScaleOff"=0.0}, {"18A70017", "Frame"="IP2\ndatabase", "NameShort"="IP2FuelClogWarn", "StartBit"=52, "NumBits"=2, "Min"=0.0, "Max"=3.0, "ScaleFac"=1.0, "ScaleOff"=0.0}, {"18A70017", "Frame"="IP2\ndatabase", "NameShort"="IP2FuelGauge", "StartBit"=56, "NumBits"=8, "Min"=0.0, "Max"=100.0, "ScaleFac"=0.4, "ScaleOff"=0.0}, {"18A70017", "Frame"="IP2\ndatabase", "NameShort"="IP2FuelWarn", "StartBit"=12, "NumBits"=2, "Min"=0.0, "Max"=3.0, "ScaleFac"=1.0, "ScaleOff"=0.0}, {"18A70017", "Frame"="IP2\ndatabase", "NameShort"="IP2GearNSig", "StartBit"=16, "NumBits"=2, "Min"=0.0, "Max"=3.0, "ScaleFac"=1.0, "ScaleOff"=0.0}, {"18A70017", "Frame"="IP2\ndatabase", "NameShort"="IP2GearRSig", "StartBit"=18, "NumBits"=2, "Min"=0.0, "Max"=3.0, "ScaleFac"=1.0, "ScaleOff"=0.0}, {"18A70017", "Frame"="IP2\ndatabase", "NameShort"="IP2HandBrkStat", "StartBit"=38, "NumBits"=2, "Min"=0.0, "Max"=3.0, "ScaleFac"=1.0, "ScaleOff"=0.0}, {"18A70017", "Frame"="IP2\ndatabase", "NameShort"="IP2HeaterStat", "StartBit"=44, "NumBits"=2, "Min"=0.0, "Max"=3.0, "ScaleFac"=1.0, "ScaleOff"=0.0}, {"18A70017", "Frame"="IP2\ndatabase", "NameShort"="IP2HighBeamSig", "StartBit"=30, "NumBits"=2, "Min"=0.0, "Max"=3.0, "ScaleFac"=1.0, "ScaleOff"=0.0}, {"18A70017", "Frame"="IP2\ndatabase", "NameShort"="IP2HornSig", "StartBit"=24, "NumBits"=2, "Min"=0.0, "Max"=0.0, "ScaleFac"=1.0, "ScaleOff"=0.0}, {"18A70017", "Frame"="IP2\ndatabase", "NameShort"="IP2LeftTurnSig", "StartBit"=32, "NumBits"=2, "Min"=0.0, "Max"=3.0, "ScaleFac"=1.0, "ScaleOff"=0.0}, {"18A70017", "Frame"="IP2\ndatabase", "NameShort"="IP2LowBeamSig", "StartBit"=28, "NumBits"=2, "Min"=0.0, "Max"=3.0, "ScaleFac"=1.0, "ScaleOff"=0.0}, {"18A70017", "Frame"="IP2\ndatabase", "NameShort"="IP2LowWaterLvlWarn", "StartBit"=6, "NumBits"=2, "Min"=0.0, "Max"=3.0, "ScaleFac"=1.0, "ScaleOff"=0.0}, {"18A70017", "Frame"="IP2\ndatabase", "NameShort"="IP2MidDoorSig", "StartBit"=22, "NumBits"=2, "Min"=0.0, "Max"=3.0, "ScaleFac"=1.0, "ScaleOff"=0.0}, {"18A70017", "Frame"="IP2\ndatabase", "NameShort"="IP2OilFilterClogWarn", "StartBit"=50, "NumBits"=2, "Min"=0.0, "Max"=3.0, "ScaleFac"=1.0, "ScaleOff"=0.0}, {"18A70017", "Frame"="IP2\ndatabase", "NameShort"="IP2RegenLeverStat", "StartBit"=40, "NumBits"=2, "Min"=0.0, "Max"=3.0, "ScaleFac"=1.0, "ScaleOff"=0.0}, {"18A70017", "Frame"="IP2\ndatabase", "NameShort"="IP2RegenOverheatWarn", "StartBit"=46, "NumBits"=2, "Min"=0.0, "Max"=3.0, "ScaleFac"=1.0, "ScaleOff"=0.0}, {"18A70017", "Frame"="IP2\ndatabase", "NameShort"="IP2RightTurnSig", "StartBit"=34, "NumBits"=2, "Min"=0.0, "Max"=3.0, "ScaleFac"=1.0, "ScaleOff"=0.0}, {"18A70017", "Frame"="IP2\ndatabase", "NameShort"="IP2SmokeDetectorWarn", "StartBit"=48, "NumBits"=2, "Min"=0.0, "Max"=3.0, "ScaleFac"=1.0, "ScaleOff"=0.0}, {"18A70017", "Frame"="IP2\ndatabase", "NameShort"="IP2ThrottleInterlockWarn", "StartBit"=0, "NumBits"=2, "Min"=0.0, "Max"=3.0, "ScaleFac"=1.0, "ScaleOff"=0.0}, {"18FEC117", "Frame"="IPMileage\ndatabase", "NameShort"="IPMileageTotalOdometer", "StartBit"=0, "NumBits"=32, "Min"=0.0, "Max"=21055406.0, "ScaleFac"=0.005, "ScaleOff"=0.0}, {"18FEC117", "Frame"="IPMileage\ndatabase", "NameShort"="IPMileageTripA", "StartBit"=32, "NumBits"=32, "Min"=0.0, "Max"=21055406.0, "ScaleFac"=0.005, "ScaleOff"=0.0}, {"18F746E6", "Frame"="InsulationTesterS\ndatabase", "NameShort"="InsulatTesterSDetailedErrCode", "StartBit"=40, "NumBits"=8, "Min"=0.0, "Max"=255.0, "ScaleFac"=1.0, "ScaleOff"=0.0}, {"18F746E6", "Frame"="InsulationTesterS\ndatabase", "NameShort"="InsulatTesterSDeviceFailure", "StartBit"=53, "NumBits"=1, "Min"=0.0, "Max"=1.0, "ScaleFac"=1.0, "ScaleOff"=0.0}, {"18F746E6", "Frame"="InsulationTesterS\ndatabase", "NameShort"="InsulatTesterSHVLeakAlertLv", "StartBit"=0, "NumBits"=3, "Min"=0.0, "Max"=7.0, "ScaleFac"=1.0, "ScaleOff"=0.0}, {"18F746E6", "Frame"="InsulationTesterS\ndatabase", "NameShort"="InsulatTesterSHVNegInsultErr", "StartBit"=51, "NumBits"=1, "Min"=0.0, "Max"=1.0, "ScaleFac"=1.0, "ScaleOff"=0.0}, {"18F746E6", "Frame"="InsulationTesterS\ndatabase", "NameShort"="InsulatTesterSHVPosInsltErr", "StartBit"=50, "NumBits"=1, "Min"=0.0, "Max"=1.0, "ScaleFac"=1.0, "ScaleOff"=0.0}, {"18F746E6", "Frame"="InsulationTesterS\ndatabase", "NameShort"="InsulatTesterSLife", "StartBit"=56, "NumBits"=8, "Min"=0.0, "Max"=255.0, "ScaleFac"=1.0, "ScaleOff"=0.0}, {"18F746E6", "Frame"="InsulationTesterS\ndatabase", "NameShort"="InsulatTesterSLv1Alert", "StartBit"=48, "NumBits"=1, "Min"=0.0, "Max"=1.0, "ScaleFac"=1.0, "ScaleOff"=0.0}, {"18F746E6", "Frame"="InsulationTesterS\ndatabase", "NameShort"="InsulatTesterSLv2Alert", "StartBit"=49, "NumBits"=1, "Min"=0.0, "Max"=1.0, "ScaleFac"=1.0, "ScaleOff"=0.0}, {"18F746E6", "Frame"="InsulationTesterS\ndatabase", "NameShort"="InsulatTesterSNegInsulatResist", "StartBit"=24, "NumBits"=16, "Min"=0.0, "Max"=65535.0, "ScaleFac"=1.0, "ScaleOff"=0.0}, {"18F746E6", "Frame"="InsulationTesterS\ndatabase", "NameShort"="InsulatTesterSPosInsulatResist", "StartBit"=8, "NumBits"=16, "Min"=0.0, "Max"=65535.0, "ScaleFac"=1.0, "ScaleOff"=0.0}, {"18F746E6", "Frame"="InsulationTesterS\ndatabase", "NameShort"="InsulatTesterSWiringFailure", "StartBit"=52, "NumBits"=1, "Min"=0.0, "Max"=1.0, "ScaleFac"=1.0, "ScaleOff"=0.0}, {"18F11FF0", "Frame"="MCU1ElectricalStat\ndatabase", "NameShort"="MCU1CANBusConnectStat", "StartBit"=52, "NumBits"=1, "Min"=0.0, "Max"=1.0, "ScaleFac"=1.0, "ScaleOff"=0.0}, {"18F11FF0", "Frame"="MCU1ElectricalStat\ndatabase", "NameShort"="MCU1HPINCurr", "StartBit"=16, "NumBits"=16, "Min"=-1000.0, "Max"=1000.0, "ScaleFac"=0.1, "ScaleOff"=-1000.0}, {"18F11FF0", "Frame"="MCU1ElectricalStat\ndatabase", "NameShort"="MCU1HPINOvercurrErr", "StartBit"=43, "NumBits"=1, "Min"=0.0, "Max"=1.0, "ScaleFac"=1.0, "ScaleOff"=0.0}, {"18F11FF0", "Frame"="MCU1ElectricalStat\ndatabase", "NameShort"="MCU1HPINOvervoltErr", "StartBit"=40, "NumBits"=1, "Min"=0.0, "Max"=1.0, "ScaleFac"=1.0, "ScaleOff"=0.0}, {"18F11FF0", "Frame"="MCU1ElectricalStat\ndatabase", "NameShort"="MCU1HPINUndervoltErr", "StartBit"=44, "NumBits"=1, "Min"=0.0, "Max"=1.0, "ScaleFac"=1.0, "ScaleOff"=0.0}, {"18F11FF0", "Frame"="MCU1ElectricalStat\ndatabase", "NameShort"="MCU1HPINVolt", "StartBit"=0, "NumBits"=16, "Min"=0.0, "Max"=1000.0, "ScaleFac"=0.1, "ScaleOff"=0.0}, {"18F11FF0", "Frame"="MCU1ElectricalStat\ndatabase", "NameShort"="MCU1HVBattConnectStat", "StartBit"=55, "NumBits"=1, "Min"=0.0, "Max"=1.0, "ScaleFac"=1.0, "ScaleOff"=0.0}, {"18F11FF0", "Frame"="MCU1ElectricalStat\ndatabase", "NameShort"="MCU1HillStartStat", "StartBit"=39, "NumBits"=1, "Min"=0.0, "Max"=1.0, "ScaleFac"=1.0, "ScaleOff"=0.0}, {"18F11FF0", "Frame"="MCU1ElectricalStat\ndatabase", "NameShort"="MCU1KeyIgniteStat", "StartBit"=54, "NumBits"=1, "Min"=0.0, "Max"=1.0, "ScaleFac"=1.0, "ScaleOff"=0.0}, {"18F11FF0", "Frame"="MCU1ElectricalStat\ndatabase", "NameShort"="MCU1LVDCPowErr", "StartBit"=53, "NumBits"=1, "Min"=0.0, "Max"=1.0, "ScaleFac"=1.0, "ScaleOff"=0.0}, {"18F11FF0", "Frame"="MCU1ElectricalStat\ndatabase", "NameShort"="MCU1Life", "StartBit"=60, "NumBits"=4, "Min"=0.0, "Max"=15.0, "ScaleFac"=1.0, "ScaleOff"=0.0}, {"18F11FF0", "Frame"="MCU1ElectricalStat\ndatabase", "NameShort"="MCU1MCUErr", "StartBit"=33, "NumBits"=1, "Min"=0.0, "Max"=1.0, "ScaleFac"=1.0, "ScaleOff"=0.0}, {"18F11FF0", "Frame"="MCU1ElectricalStat\ndatabase", "NameShort"="MCU1McuOverheatErr", "StartBit"=46, "NumBits"=1, "Min"=0.0, "Max"=1.0, "ScaleFac"=1.0, "ScaleOff"=0.0}, {"18F11FF0", "Frame"="MCU1ElectricalStat\ndatabase", "NameShort"="MCU1McuTempAlert", "StartBit"=51, "NumBits"=1, "Min"=0.0, "Max"=1.0, "ScaleFac"=1.0, "ScaleOff"=0.0}, {"18F11FF0", "Frame"="MCU1ElectricalStat\ndatabase", "NameShort"="MCU1Mode", "StartBit"=34, "NumBits"=5, "Min"=0.0, "Max"=31.0, "ScaleFac"=1.0, "ScaleOff"=0.0}, {"18F11FF0", "Frame"="MCU1ElectricalStat\ndatabase", "NameShort"="MCU1MtrOverheatErr", "StartBit"=45, "NumBits"=1, "Min"=0.0, "Max"=1.0, "ScaleFac"=1.0, "ScaleOff"=0.0}, {"18F11FF0", "Frame"="MCU1ElectricalStat\ndatabase", "NameShort"="MCU1MtrOverspdErr", "StartBit"=47, "NumBits"=1, "Min"=0.0, "Max"=1.0, "ScaleFac"=1.0, "ScaleOff"=0.0}, {"18F11FF0", "Frame"="MCU1ElectricalStat\ndatabase", "NameShort"="MCU1MtrPosnSensorErr", "StartBit"=42, "NumBits"=1, "Min"=0.0, "Max"=1.0, "ScaleFac"=1.0, "ScaleOff"=0.0}, {"18F11FF0", "Frame"="MCU1ElectricalStat\ndatabase", "NameShort"="MCU1MtrTempAlert", "StartBit"=50, "NumBits"=1, "Min"=0.0, "Max"=1.0, "ScaleFac"=1.0, "ScaleOff"=0.0}, {"18F11FF0", "Frame"="MCU1ElectricalStat\ndatabase", "NameShort"="MCU1NoPermsToOp", "StartBit"=57, "NumBits"=1, "Min"=0.0, "Max"=1.0, "ScaleFac"=1.0, "ScaleOff"=0.0}, {"18F11FF0", "Frame"="MCU1ElectricalStat\ndatabase", "NameShort"="MCU1PermsToOp", "StartBit"=56, "NumBits"=1, "Min"=0.0, "Max"=1.0, "ScaleFac"=1.0, "ScaleOff"=0.0}, {"18F11FF0", "Frame"="MCU1ElectricalStat\ndatabase", "NameShort"="MCU1PhaseCurrErr", "StartBit"=32, "NumBits"=1, "Min"=0.0, "Max"=1.0, "ScaleFac"=1.0, "ScaleOff"=0.0}, {"18F11FF0", "Frame"="MCU1ElectricalStat\ndatabase", "NameShort"="MCU1PhaseUOvercurrErr", "StartBit"=48, "NumBits"=1, "Min"=0.0, "Max"=1.0, "ScaleFac"=1.0, "ScaleOff"=0.0}, {"18F11FF0", "Frame"="MCU1ElectricalStat\ndatabase", "NameShort"="MCU1PhaseWOvercurrErr", "StartBit"=49, "NumBits"=1, "Min"=0.0, "Max"=1.0, "ScaleFac"=1.0, "ScaleOff"=0.0}, {"18F120F0", "Frame"="MCU2MtrStat\ndatabase", "NameShort"="MCU2CurrentMtrRPM", "StartBit"=16, "NumBits"=16, "Min"=-12000.0, "Max"=12000.0, "ScaleFac"=1.0, "ScaleOff"=-12000.0}, {"18F120F0", "Frame"="MCU2MtrStat\ndatabase", "NameShort"="MCU2McuTemp", "StartBit"=56, "NumBits"=8, "Min"=-40.0, "Max"=210.0, "ScaleFac"=1.0, "ScaleOff"=-40.0}, {"18F120F0", "Frame"="MCU2MtrStat\ndatabase", "NameShort"="MCU2MtrActualTorq", "StartBit"=32, "NumBits"=16, "Min"=-3000.0, "Max"=3000.0, "ScaleFac"=0.1, "ScaleOff"=-3000.0}, {"18F120F0", "Frame"="MCU2MtrStat\ndatabase", "NameShort"="MCU2MtrPeakTorq", "StartBit"=0, "NumBits"=16, "Min"=-3000.0, "Max"=3000.0, "ScaleFac"=0.1, "ScaleOff"=-3000.0}, {"18F120F0", "Frame"="MCU2MtrStat\ndatabase", "NameShort"="MCU2MtrTemp", "StartBit"=48, "NumBits"=8, "Min"=-40.0, "Max"=210.0, "ScaleFac"=1.0, "ScaleOff"=-40.0}, {"18F121F0", "Frame"="MCU3ErrorStat\ndatabase", "NameShort"="MCU3DriveshaftTorq", "StartBit"=48, "NumBits"=16, "Min"=-3000.0, "Max"=3000.0, "ScaleFac"=0.1, "ScaleOff"=-3000.0}, {"18F121F0", "Frame"="MCU3ErrorStat\ndatabase", "NameShort"="MCU3ErrCode", "StartBit"=8, "NumBits"=8, "Min"=0.0, "Max"=255.0, "ScaleFac"=1.0, "ScaleOff"=0.0}, {"18F121F0", "Frame"="MCU3ErrorStat\ndatabase", "NameShort"="MCU3ErrLv", "StartBit"=4, "NumBits"=4, "Min"=0.0, "Max"=4.0, "ScaleFac"=1.0, "ScaleOff"=0.0}, {"18F121F0", "Frame"="MCU3ErrorStat\ndatabase", "NameShort"="MCU3HwVer", "StartBit"=27, "NumBits"=5, "Min"=0.0, "Max"=31.0, "ScaleFac"=1.0, "ScaleOff"=0.0}, {"18F121F0", "Frame"="MCU3ErrorStat\ndatabase", "NameShort"="MCU3SwVer", "StartBit"=16, "NumBits"=11, "Min"=0.0, "Max"=2047.0, "ScaleFac"=1.0, "ScaleOff"=0.0}, {"18F121F0", "Frame"="MCU3ErrorStat\ndatabase", "NameShort"="MCU3SysStat", "StartBit"=0, "NumBits"=4, "Min"=0.0, "Max"=6.0, "ScaleFac"=1.0, "ScaleOff"=0.0}, {"1FFFFFFC", "Frame"="PCINPUT\ndatabase", "NameShort"="PCRXMsg1", "StartBit"=0, "NumBits"=16, "Min"=0.0, "Max"=65.535, "ScaleFac"=0.001, "ScaleOff"=0.0}, {"1FFFFFFC", "Frame"="PCINPUT\ndatabase", "NameShort"="PCRXMsg3", "StartBit"=16, "NumBits"=16, "Min"=0.0, "Max"=65.535, "ScaleFac"=0.001, "ScaleOff"=0.0}, {"1FFFFFFC", "Frame"="PCINPUT\ndatabase", "NameShort"="PCRXMsg5", "StartBit"=32, "NumBits"=16, 
